vi "jsonKey.vi"(8 "error in (no error)":errorcluster, 9 "index":i32, 10 "path":string, 11 "d in":i64) -> (0 "error out":errorcluster, 2 "key":string, 3 "d out":i64)   [LabVIEW 2015, in "JSON Document.lvclass"]
uses:
  API/JSON Document Class/JSON Document.lvclass
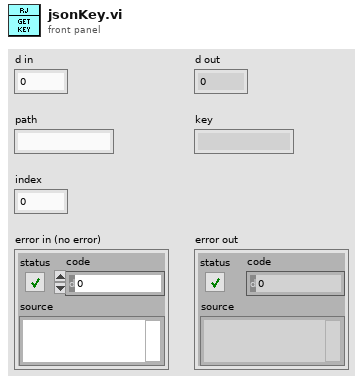
[diagram p1: front panel]
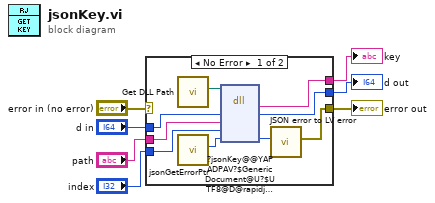
[diagram p0: block diagram]
diagram:
  n1 = case shown="No Error" "error in (no error)" {
    selector: "error in (no error)" -> [_ w18]
    tunnel: [w13 w18] -> w7
    tunnel: "d in" -> [w12 w17]
    tunnel: [w11 w17] -> w4
    tunnel: "path" -> [w10 _]
    tunnel: [w9 _] -> w2
    tunnel: "index" -> [w8 _]
    frame No Error {
      n2 = call "Get DLL Path.vi"() -> ("Path"=w16:path)  [unwired: 11 in]
      n3 = call "jsonGetErrorPtr.vi"() -> ("return type"=w15:i64)  [unwired: 10 in, 1 out]
      n4 = dll-call lib="C:/Users/tblair/Documents/Git Projects/rapidjson-for-LabVIEW/lvrjs/Debug/lvrjs.dll" fn="?jsonKey@@YAPADPAV?$GenericDocument@U?$UTF8@D@rapidjson@@V?$MemoryPoolAllocator@VCrtAllocator@rapidjson@@@2@VCrtAllocator@2@@rapidjson@@PADH0@Z"(path in=w16, "d"=w12, "path"=w10, "index"=w8, "jsonError"=w15) -> ("return type"=w9:string, "d"=w11:i64, "jsonError"=w14:i64)  [unwired: 4 in, 2 out]
      n5 = call "JSON error to LV error.vi"("jsonError"=w14) -> ("error out"=w13:errorcluster)  [unwired: 10 in]
    }
    frame Error {
    }
  }
  "error out" <- w7
  "d out" <- w4
  "key" <- w2
